vi "VTxIndex_control.vi"(4 "Unfreeze":bool, 6 "Is_D_mode":bool, 7 "VTx1_volt":dbl=90.0, 8 "error in (no error)":errorcluster, 9 "Timeout (ms)":i32=40000000, 10 "VTxIndex_In":i8, 11 "connection ID in":refnum<k5>) -> (0 "error out":errorcluster, 2 "VTxIndex_Out":i8, 3 "connection ID out":refnum<k5>)   [LabVIEW 2016]
uses:
  TemperatureMeasure/Thermal_type.vi
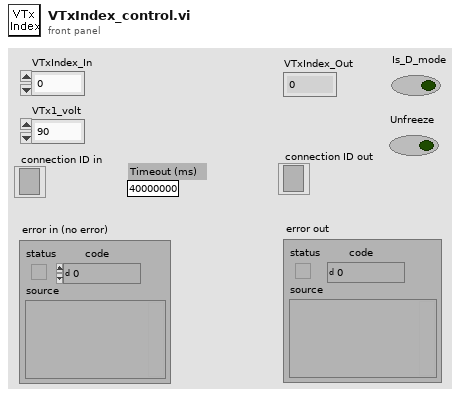
[diagram p1: front panel]
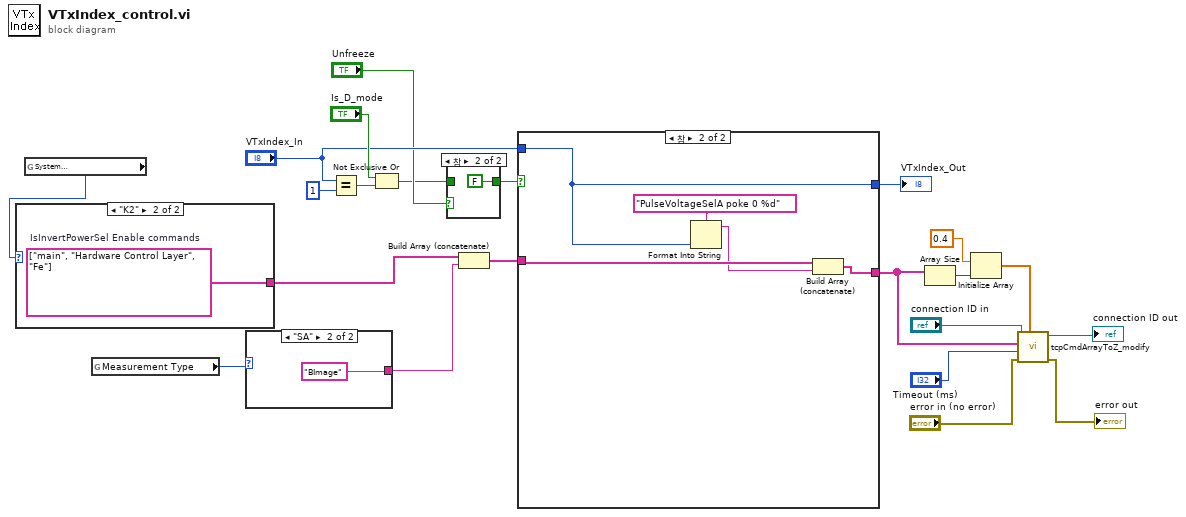
[diagram p0: block diagram]
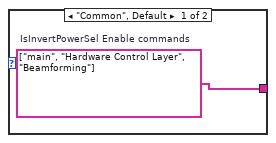
[diagram p2: hidden frame]
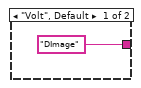
[diagram p3: hidden frame]
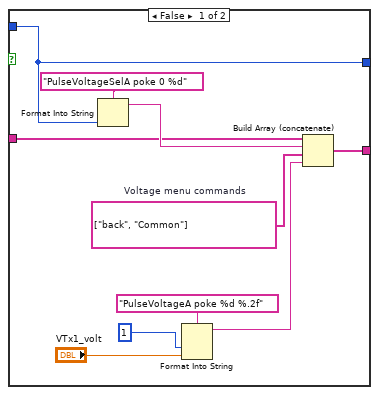
[diagram p5: hidden frame]
diagram:
  n1 = global read "Thermal_type.vi" "System \nSelection"() -> (w1:enum32{"Common", "Frosk", "Griffin", "K2"})
  n2 = case shown="\"K2\"" w1 {
    tunnel: [w23 w24] -> w4
    frame "Common", Default {
      w23 = string[] ["main", "Hardware Control Layer", "Beamforming"]  # IsInvertPowerSel Enable commands
    }
    frame "K2" {
      w24 = string[] ["main", "Hardware Control Layer", "Fe"]  # IsInvertPowerSel Enable commands
    }
  }
  n3 = global read "Thermal_type.vi" "Measurement Type"() -> (w5:enum32{"Volt", "SA"})
  n4 = case shown="\"SA\"" w5 {
    tunnel: ["DImage" "BImage"] -> w3
    frame "Volt", Default {
    }
    frame "SA" {
    }
  }
  n5 = Equal?(x="VTxIndex_In", y=i8 1) -> (x = y?=w9:bool)
  n6 = Not Exclusive Or(1:w9, 2:"Is_D_mode") -> (0:w6:bool)
  n7 = case shown="참" "Unfreeze" {
    tunnel: [w27 FALSE] -> w7
    tunnel: w6 -> [w27 _]
    frame False {
    }
    frame True {
    }
  }
  n8 = Build Array (concatenate)(w4, w3) -> (w2:string[])
  n9 = case shown="참" w7 {
    tunnel: [w29 w39] -> w22
    tunnel: w2 -> [w36 w43]
    tunnel: [w30 w42] -> w13
    tunnel: "VTxIndex_In" -> [w29 w39]
    frame False {
      w32 = string[] ["back", "Common"]  # Voltage menu commands
      n10 = Format Into String(format string="PulseVoltageSelA poke 0 %d" ("포맷 문자열"), w29) -> (resulting string=w38:string)  [unwired: 2 in, 1 out]
      n11 = Format Into String(format string="PulseVoltageA poke %d %.2f" ("Format String"), i8 1 ("input 1"), "VTx1_volt") -> (resulting string=w31:string)  [unwired: 2 in, 1 out]
      n12 = Build Array (concatenate)(w36, w38, w32, w31) -> (w30:string[])
    }
    frame True {
      n13 = Format Into String(format string="PulseVoltageSelA poke 0 %d" ("포맷 문자열"), w39) -> (resulting string=w40:string)  [unwired: 2 in, 1 out]
      n14 = Build Array (concatenate)(w43, w40) -> (w42:string[])
    }
  }
  "VTxIndex_Out" <- w22
  n15 = Array Size(array=w13) -> (size(s)=w21:i32)
  n16 = Initialize Array(0.4 ("원소"), w21) -> (w14:dbl[])
  n17 = call "tcpCmdArrayToZ_modify.vi"("Delay (sec)"=w14, "error in (no error)"="error in (no error)", "Timeout (ms)"="Timeout (ms)", "Command array"=w13, "connection ID in"="connection ID in") -> ("error out"=→"error out":errorcluster, "connection ID out"=→"connection ID out":refnum<k5>)  [unwired: 2 in, 3 out]
